vi "ReadWrite.Initialize.vi"(8 "error in (no error)":errorcluster, 11 "ReadWrite in":refnum<class "ReadWrite.lvclass">) -> (0 "error out":errorcluster, 3 "ReadWrite out":refnum<class "ReadWrite.lvclass">)   [LabVIEW 2015, in "Data Access API.lvlib" / "ReadWrite.lvclass"]
uses:
  ReadWrite.lvclass
  ReadWrite.lvclass/ReadWrite.ctl
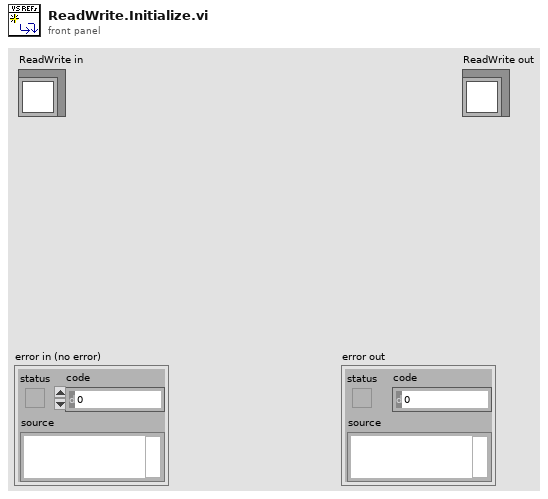
[diagram p1: front panel]
types:
  T1 = cluster{"read mode":enum16{"polling", "blocking"}, "write mode":enum16{"polling", "blocking"}}
  T2 = typedef "Custom Device API.lvlib/Data Reference.ctl" = i32
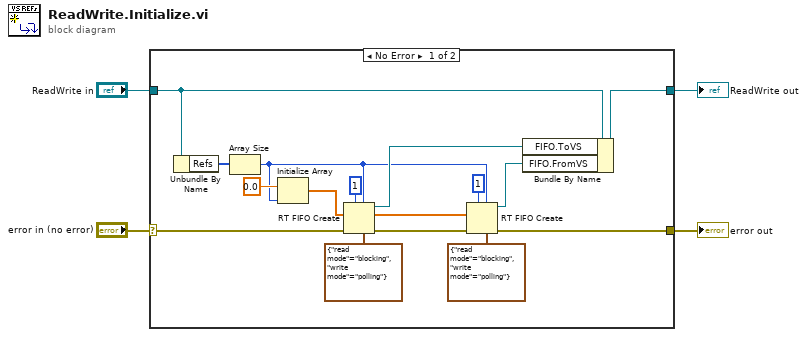
[diagram p0: block diagram]
diagram:
  n1 = case shown="No Error" "error in (no error)" {
    selector: "error in (no error)" -> [w5 w21]
    tunnel: [w12 w21] -> w4
    tunnel: "ReadWrite in" -> [w7 w20]
    tunnel: [w6 w20] -> w2
    frame No Error {
      n2 = Unbundle By Name(w7) -> ("Refs"=w8:T2[])
      n3 = Array Size(array=w8) -> (size(s)=w11:i32)
      n4 = Initialize Array(0.0 ("element"), w11) -> (w10:dbl[])
      n5 = RT FIFO Create(1:w10, 3:w5, 4:u32 1 ("size (10)"), 6:w11, 7:T1 {"read mode"=enum."blocking", "write mode"=enum."polling"} ("r/w modes (polling,polling)")) -> (8:w18:refnum<k33>, 11:w9:errorcluster)  [unwired: 3 in, 1 out]
      n6 = RT FIFO Create(1:w10, 3:w9, 4:u32 1 ("size (10)"), 6:w11, 7:T1 {"read mode"=enum."blocking", "write mode"=enum."polling"} ("r/w modes (polling,polling)")) -> (8:w19:refnum<k33>, 11:w12:errorcluster)  [unwired: 3 in, 1 out]
      n7 = Bundle By Name(cluster=w7, "FIFO.ToVS"=w18, "FIFO.FromVS"=w19) -> (w6:refnum<class "ReadWrite.lvclass">)
    }
    frame Error {
    }
  }
  "error out" <- w4
  "ReadWrite out" <- w2
